vi "DC Supply Init.vi"(8 "error in":errorcluster, 9 "Reset (F:no)":bool, 11 "VISA resource name":refnum<visa-resource-name>) -> (0 "error out":errorcluster, 3 "VISA resource name out":refnum<visa-resource-name>)   [LabVIEW 2019, in "DAC.lvlib" / "DAC DC Supply.lvclass"]
uses:
  DAC DC Supply.lvclass
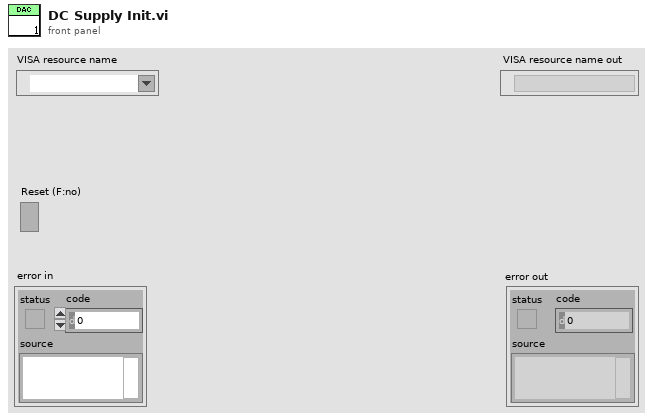
[diagram p1: front panel]
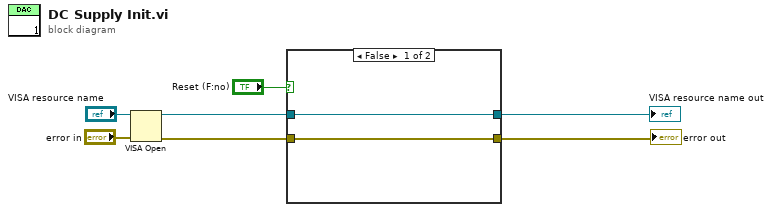
[diagram p0: block diagram]
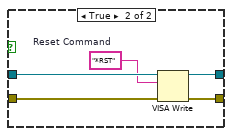
[diagram p2: hidden frame]
diagram:
  n1 = VISA Open(error in (no error)="error in", VISA resource name="VISA resource name") -> (VISA resource name=w3:refnum<visa-resource-name>, error out=w2:errorcluster)  [unwired: 3 in]
  n2 = case shown="False" "Reset (F:no)" {
    tunnel: w2 -> [w9 w12]
    tunnel: [w9 w10] -> w1
    tunnel: w3 -> [w8 w14]
    tunnel: [w8 w11] -> w5
    frame False {
    }
    frame True {
      w13 = "*RST"  # Reset Command
      n3 = VISA Write(VISA resource name=w14, write buffer=w13, error in (no error)=w12) -> (VISA resource name out=w11:refnum<visa-resource-name>, error out=w10:errorcluster)  [unwired: 1 out]
    }
  }
  "VISA resource name out" <- w5
  "error out" <- w1
